vi "UUT - Play tone.vi"(8 "error in (no error)":errorcluster, 10 "Frequency":dbl, 11 "VISA resource name":refnum<visa-resource-name>) -> (0 "error out":errorcluster, 3 "VISA resource name out":refnum<visa-resource-name>)   [LabVIEW 2011]
uses:
  Audio Hardware Simulation Commands.ctl
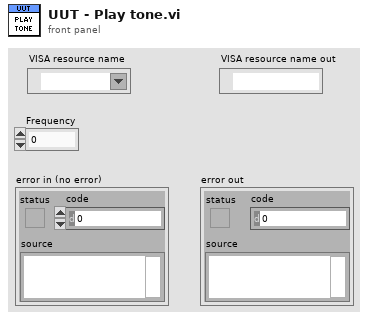
[diagram p1: front panel]
types:
  T1 = typedef "Audio Hardware Simulation Commands.ctl" = enum16{"Simulate Play Waveform", "Mic Test - Simulate Read Microphone", "Spkr Test - Simulate Read Microphone"}
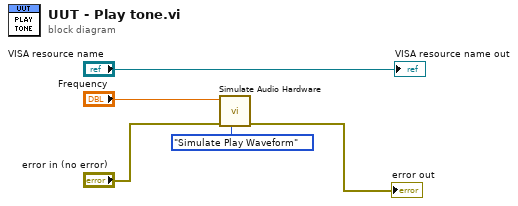
[diagram p0: block diagram]
diagram:
  n1 = call "Simulate Audio Hardware.vi"("Command to Simulate"=Audio_Hardware_Simulation_Commands."Simulate Play Waveform", "error in (no error)"="error in (no error)", "Frequency"="Frequency") -> ("error out"=→"error out":errorcluster)  [unwired: 6 in, 1 out]
  "VISA resource name out" <- "VISA resource name"
